vi "Listen.vi"(8 "error in (no error)":errorcluster caption="entrée d'erreur (pas d'erreur)", 11 "Server TCP_IP (Default) en entrée":refnum<class "Server TCP_IP (Default).lvclass">) -> (0 "error out":errorcluster caption="sortie d'erreur", 3 "Server TCP_IP (Default) en sortie":refnum<class "Server TCP_IP (Default).lvclass">)   [LabVIEW 2020, in "Library Instrument & Equipement.lvlib" / "Library TCP IP.lvlib" / "Server TCP_IP (Default).lvclass"]
uses:
  Server TCP_IP (Default).lvclass
  Server TCP_IP (Default).lvclass/Server TCP_IP (Default).ctl
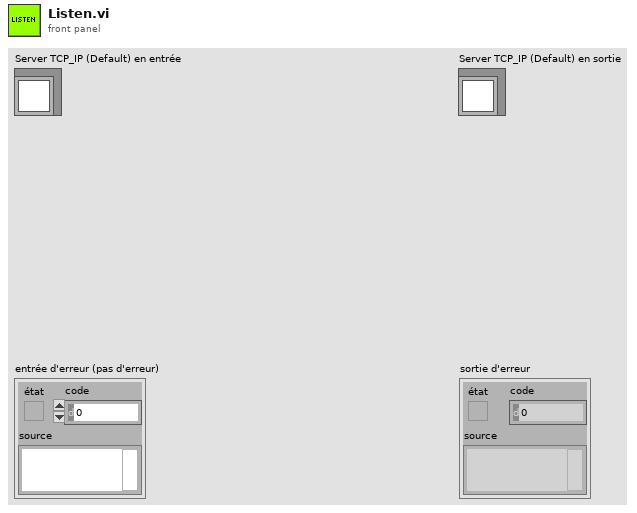
[diagram p1: front panel]
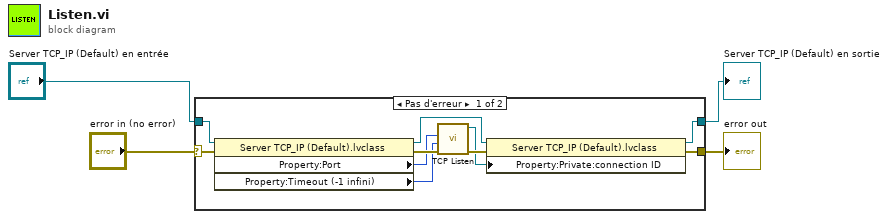
[diagram p0: block diagram]
diagram:
  n1 = case shown="Pas d'erreur" "error in (no error)" {
    selector: "error in (no error)" -> [w5 w16]
    tunnel: [w12 w16] -> w3
    tunnel: [w6 w15] -> w1
    tunnel: "Server TCP_IP (Default) en entrée" -> [w14 w15]
    frame No Error {
      n2 = property class="Server TCP_IP (Default).lvclass"(reference=w14, error in=w5) -> (reference out=w13:refnum<class "Server TCP_IP (Default).lvclass">, error out=w10:errorcluster, "Property:Port"=w8:i16, "Property:Timeout (-1 infini)"=w7:i16)
      n3 = call <vilib>:"TCP Listen.vi"("error in (no error)"=w10, "timeout ms (wait forever: -1)"=w7, "port"=w8) -> ("error out"=w11:errorcluster, "connection ID"=w9:refnum<k5>)  [unwired: 4 in, 3 out]
      n4 = property class="Server TCP_IP (Default).lvclass"(reference=w13, error in=w11, "Property:Private:connection ID"=w9) -> (reference out=w6:refnum<class "Server TCP_IP (Default).lvclass">, error out=w12:errorcluster)
    }
    frame Error {
    }
  }
  "error out" <- w3
  "Server TCP_IP (Default) en sortie" <- w1
